vi "Elapsed Times Graph.vi"(3 "User Identification:":string) -> ()   [LabVIEW 2011]
doc: "This graphs the elapsed time between calls.\nIt is used to measure how long events or code are taking."
panel:
  out "Called From:":string
  out "Elapsed Time":cluster{"Moving Average":dbl, dbl}(graph)
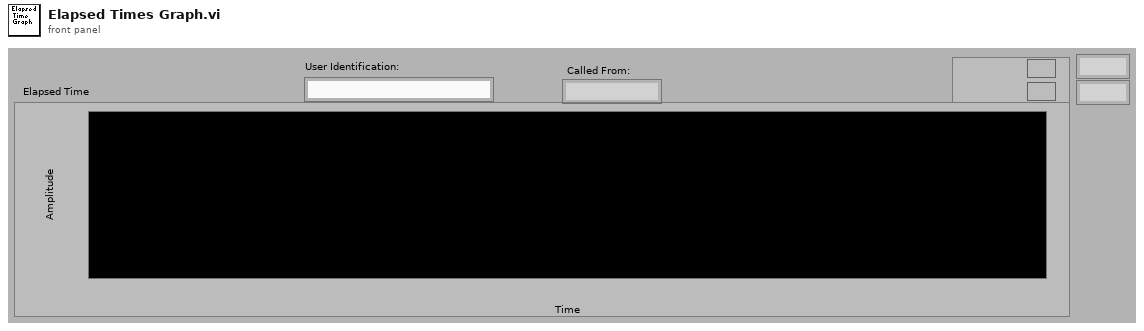
[diagram p1: front panel]
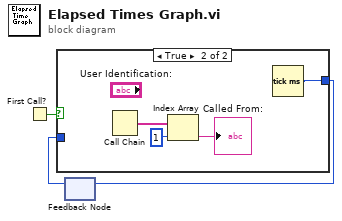
[diagram p0: block diagram]
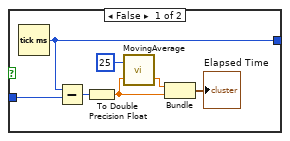
[diagram p2: hidden frame]
diagram:
  n1 = First Call?() -> (First Call?: T/F=w3:bool)
  n2 = feedback #1() -> (w1:u32)  [unwired: 1 out]
  n3 = case shown="True" w3 {
    tunnel: [w10 w14] -> w2
    tunnel: w1 -> [w9 _]
    frame False {
      n4 = Tick Count (ms)() -> (millisecond timer value=w10:u32)
      n5 = Subtract(x=w10, y=w9) -> (x-y=w5:u32)
      n6 = To Double Precision Float(number=w5) -> (double precision float=w4:dbl)
      n7 = call "MovingAverage.vi"("Additional Value"=w4, "# to Average"=25) -> ("Moving Average"=w6:dbl)  [unwired: 1 out]
      n8 = Bundle("Moving Average"=w6, w4) -> (→"Elapsed Time":cluster{"Moving Average":dbl, dbl})  [unwired: 1 out]
    }
    frame True {
      n9 = Call Chain() -> (call chain=w12:string[])
      n10 = Index Array(array=w12, index=1 ("millisecond timer value")) -> (element=→"Called From:":string)
      n11 = Tick Count (ms)() -> (millisecond timer value=w14:u32)
    }
  }
  n12 = feedback-in #1(w2) -> ()
